vi "FRC Color Processing Example.vi"(0 "Image In":T1, 2 "LED Color":T5={"Hue"={110.52399131877658, 148.6727294921875}, "Sat"={34.78571428571429, 255.0}, "Val"={91.07142857142858, 255.0}} {"Hue" scale=0.0..255.0 scale format="%#_3g"}, 4 "Camera Type":T2=enum."MS HD3000 square") -> (7 "Original Image":T1(plugin-control), 9 "Detected Targets":T3(array[cluster]) {"Normalized Rect"."Numeric 5" format="%#_2g"; "Normalized Rect"."Numeric 3" format="%#_2g"; "Normalized Rect"."Numeric 2" format="%#_2g"; "Normalized Rect"."Numeric" format="%#_2g"})   [LabVIEW 2015]
uses:
  Users/allenpeters/git/Beachbot2016Dash/vision/Camera Types.ctl
  <vilib>/vision/Image Controls.llb/IMAQ Image.ctl
  <vilib>/vision/NI_Vision_Development_Module.lvlib
panel:
  in  "Std Devs for Calibration":cluster{"H":dbl, "S":dbl, "V":dbl}={"H"=4.0, "S"=6.0, "V"=6.0}
  out "Highest Avg Score":dbl format="%#_3g"
  in  "Min Score Threshold":i32=70
  in  "Emphasize Limit Tests":bool=TRUE
  in  "Aspect Ratio Fudge Factor":dbl=1.0
  in  "Annotation Limit":dbl=75.0
  in  "Annotate":bool=TRUE
  out "Sorted Particle Scores":T4(array[cluster]) {"Moment Factor" format="%#_3g"; "Aspect Ratio" format="%#_3g"; "Area to CH" format="%#_3g"; "X" format="%#_3g"; "Y" format="%#_3g"}
  out "Qualified Particles":i32
  out "Masked":T1(plugin-control)
  # "Instructions:\nUse Source to select image files from a directory, or use a USB or IP camera connected to your laptop.\nUse LED Color to threshold and build particles. Adjust HSV values to improve masking.\nClick and draw a line in Original Image to auto-calibrate to the LED color. You may need to widen Sat and Val.\nAnnotations draw a rectangle around \"good\" particles with scores from top to bottom."
  # "Density Profile"
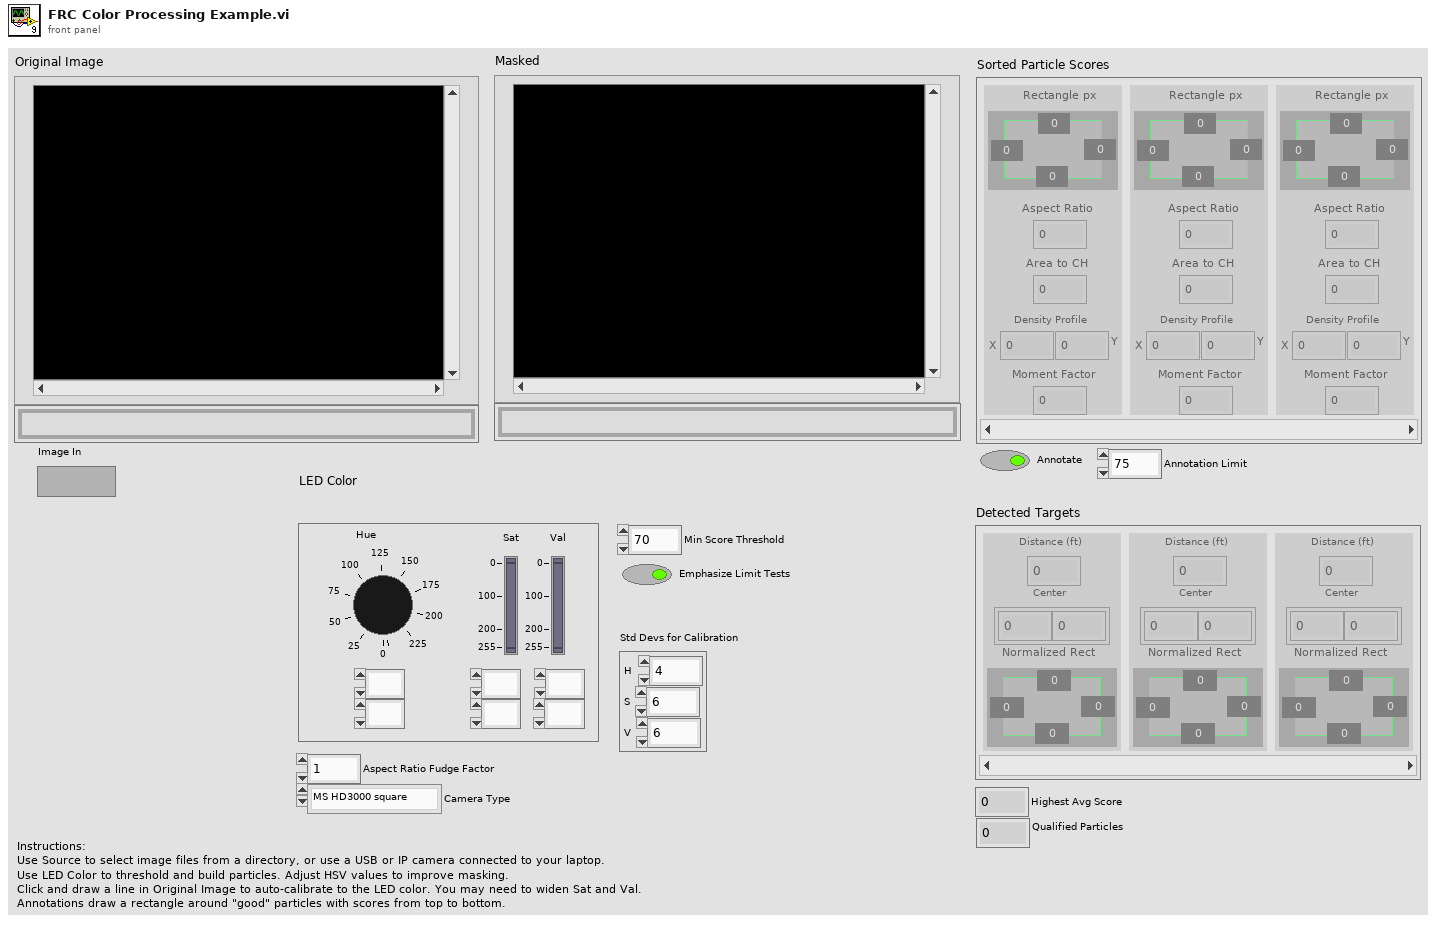
[diagram p1: front panel]
types:
  T1 = typedef "IMAQ Image.ctl" = refnum<image>
  T2 = typedef "Camera Types.ctl" = enum16{"206", "1011", "1013", "MS HD3000 square", "MS HD3000 640x480"}
  T3 = cluster{"Distance (ft)":dbl, "Center":cluster{dbl, dbl}, "Normalized Rect":cluster{"Numeric":dbl, "Numeric 2":dbl, "Numeric 3":dbl, "Numeric 5":dbl}}[]
  T4 = cluster{"Rectangle px":cluster{"Numeric":dbl, "Numeric 2":dbl, "Numeric 3":dbl, "Numeric 5":dbl}, "Aspect Ratio":dbl, "Area to CH":dbl, "X":dbl, "Y":dbl, "Moment Factor":dbl}[]
  T5 = cluster{"Hue":cluster{dbl, dbl}, "Sat":cluster{dbl, dbl}, "Val":cluster{dbl, dbl}}
  T6 = typedef "Particle Parameters" = i32
  T7 = typedef "Image Type" = u32
  T8 = cluster{cluster{dbl, dbl}, cluster{dbl, dbl}, cluster{dbl, dbl}}
  T9 = cluster{"Bounding box":cluster{"left":dbl, "top":dbl, "right":dbl, "bottom":dbl}, "Aspect Ratio":dbl, "Area to CH":dbl, "X Mask":dbl, "Y Mask":dbl, "Moment":dbl}[]
  T10 = cluster{"Rectangle":cluster{"Numeric":dbl, "Numeric 2":dbl, "Numeric 3":dbl, "Numeric 5":dbl}, "L":dbl, "Area to CH":dbl, "X":dbl, "Y":dbl, "Moment Factor":dbl}[]
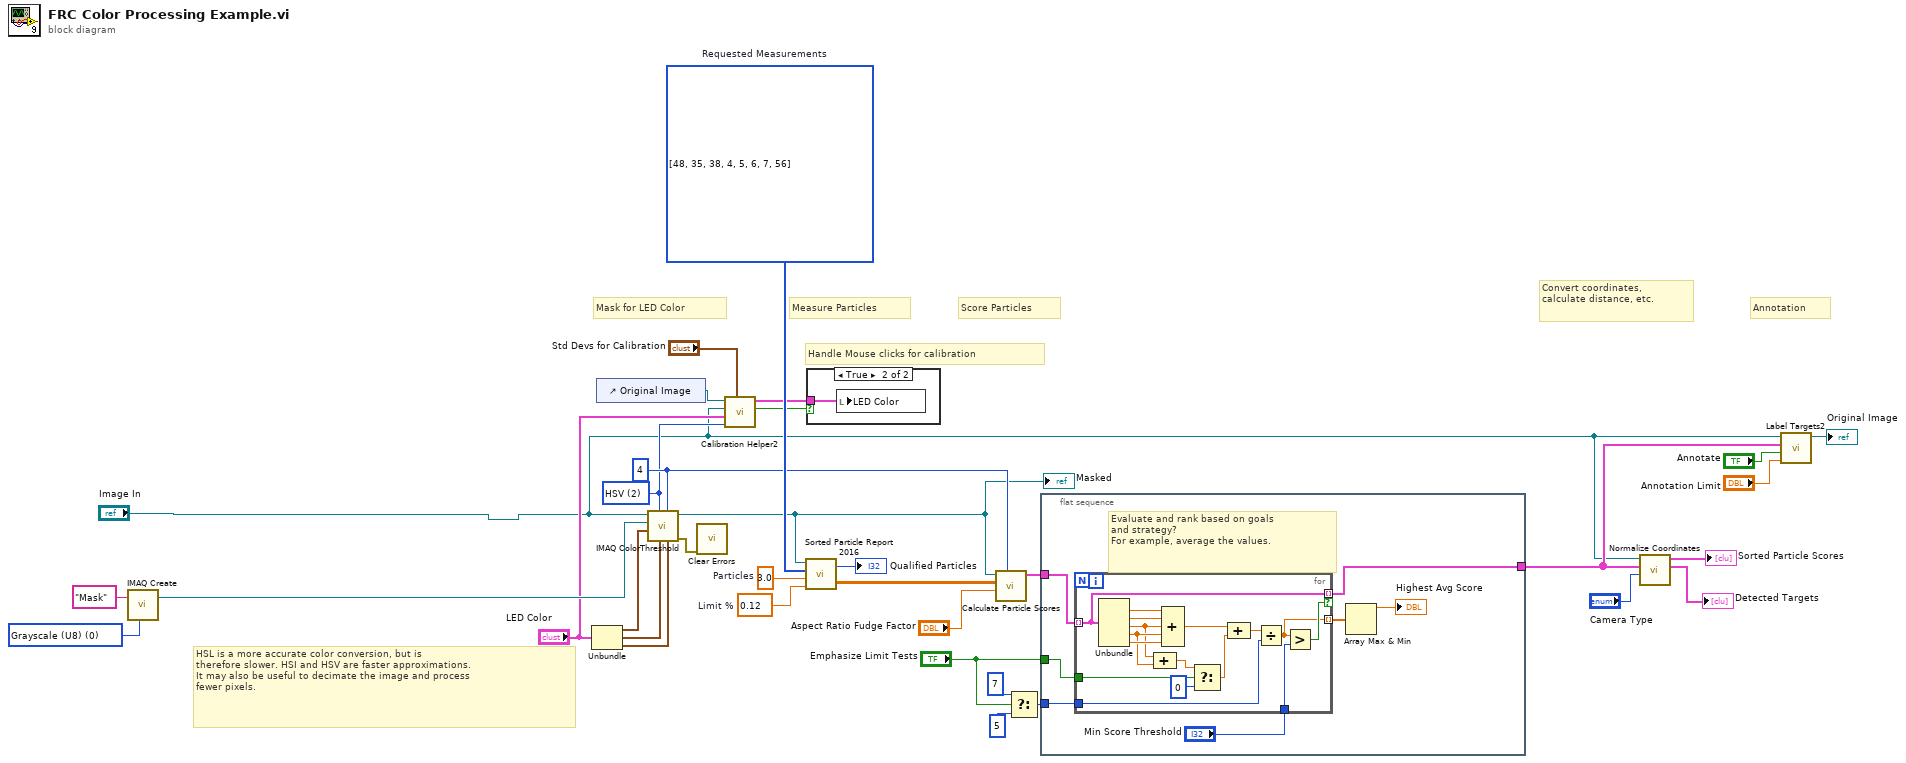
[diagram p0: block diagram]
diagram:
  w21 = 4 ("Replace Value")
  w24 = 0.12  # Limit %
  w27 = 3.0  # Particles
  w5 = u16 2 items=["RGB", "HSL", "HSV", "HSI"] ("Color Mode")
  w31 = T6[] [48, 35, 38, 4, 5, 6, 7, 56] items=["Center of Mass X", "Center of Mass Y", "First Pixel X", "First Pixel Y", "Bounding Rect Left", "Bounding Rect Top", "Bounding Rect Right", "Bounding Rect Bottom", "Max Feret Diameter Start X", "Max Feret Diameter Start Y", "Max Feret Diameter End X", "Max Feret Diameter End Y", "Max Horiz. Segment Length Left", "Max Horiz. Segment Length Right", "Max Horiz. Segment Length Row", "-", "Bounding Rect Width", "Bounding Rect Height", "Bounding Rect Diagonal", "Perimeter", "Convex Hull Perimeter", "Holes' Perimeter", "Max Feret Diameter", "Equivalent Ellipse Major Axis", "Equivalent Ellipse Minor Axis", "Equivalent Ellipse Minor Axis (Feret)", "Equivalent Rect Long Side", "Equivalent Rect Short Side", "Equivalent Rect Diagonal", "Equivalent Rect Short Side (Feret)", "Average Horiz. Segment Length", "Average Vert. Segment Length", "Hydraulic Radius", "Waddel Disk Diameter", "-", "Area", "Holes' Area", "Particle & Holes' Area", "Convex Hull Area", "Image Area", "-", "Number of Holes", "Number of Horiz. Segments", "Number of Vert. Segments", "-", "Orientation", "Max Feret Diameter Orientation", "-", "% Area/Image Area", "% Area/(Particle & Holes' Area)", "Ratio of Equivalent Ellipse Axes", "Ratio of Equivalent Rect Sides", "-", "Elongation Factor", "Compactness Factor", "Heywood Circularity Factor", "Type Factor", "-", "Sum X", "Sum Y", "Sum XX", "Sum XY", "Sum YY", "Sum XXX", "Sum XXY", "Sum XYY", "Sum YYY", "-", "Moment of Inertia XX", "Moment of Inertia XY", "Moment of Inertia YY", "Moment of Inertia XXX", "Moment of Inertia XXY", "Moment of Inertia XYY", "Moment of Inertia YYY", "Norm. Moment of Inertia XX", "Norm. Moment of Inertia XY", "Norm. Moment of Inertia YY", "Norm. Moment of Inertia XXX", "Norm. Moment of Inertia XXY", "Norm. Moment of Inertia XYY", "Norm. Moment of Inertia YYY", "Hu Moment 1", "Hu Moment 2", "Hu Moment 3", "Hu Moment 4", "Hu Moment 5", "Hu Moment 6", "Hu Moment 7"]  # Requested Measurements
  w34 = T7 0 items=["Grayscale (U8)", "Grayscale (I16)", "Grayscale (SGL)", "Complex (CSG)", "RGB (U32)", "HSL (U32)", "RGB (U64)", "Grayscale (U16)"] ("Image Type")
  # "Handle Mouse clicks for calibration"
  # "Measure Particles"
  # "Convert coordinates,\ncalculate distance, etc."
  # "Annotation"
  # "Score Particles"
  # "Mask for LED Color"
  # "HSL is a more accurate color conversion, but is\ntherefore slower. HSI and HSV are faster approximations.\nIt may also be useful to decimate the image and process\nfewer pixels."
  n1 = call "IMAQ Create"("Image Name"="Mask", "Image Type"=w34) -> ("New Image"=w32:T1)  [unwired: 2 in, 2 out]
  n2 = Unbundle("LED Color") -> ("Hue"=w30:cluster{dbl, dbl}, "Sat"=w29:cluster{dbl, dbl}, "Val"=w28:cluster{dbl, dbl})
  n3 = control-ref of="Original Image"() -> (w8:refnum<vi>)
  n4 = call "IMAQ ColorThreshold"("Blue or Luma or Val or Inten Range"=w28, "Replace Value"=w21, "Green or Sat Range"=w29, "Color Mode"=w5, "Red or Hue Range"=w30, "Image Dst"=w32, "Image Src"="Image In") -> ("error out"=w12:errorcluster, "Image Dst Out"=w13:T1)  [unwired: 3 in]
  "Masked" <- w13
  n5 = call <vilib>:"Clear Errors.vi"("error in (no error)"=w12) -> ()  [unwired: 5 in, 2 out]
  n6 = call "Calibration Helper2.vi"("Std Devs"="Std Devs for Calibration", "Color Mode"=w5, "Color Components"="LED Color", "Image"="Image In", "Image Ctl Refnum"=w8) -> ("Changed"=w7:bool, "output color"=w6:T8)  [unwired: 5 in]
  n7 = call "Sorted Particle Report 2016.vi"("Min Area Size %"=w24, "Particle Count Limit"=w27, "Pixel Measurements"=w31, "Image in"=w13) -> ("Sorted Data"=w25:dbl[][], "Particles"=→"Qualified Particles":i32)
  n8 = case shown="True" w7 {
    tunnel: w6 -> [_ w35]
    frame False {
    }
    frame True {
      n9 = local write "LED Color"(w35) -> ()
    }
  }
  n10 = call "Calculate Particle Scores.vi"("Pixel Value"=w21, "Aspect Fudge Factor"="Aspect Ratio Fudge Factor", "Sorted Data"=w25, "Image in"=w13) -> ("Scores"=w16:T9)  [unwired: 7 in]
  n11 = Select(t=7, s="Emphasize Limit Tests", f=5) -> (s? t:f=w9:i32)
  n12 = flat-sequence {
    tunnel: w16 -> [w41]
    tunnel: [w42] -> w14
    tunnel: w9 -> [w38]
    tunnel: "Emphasize Limit Tests" -> [w36]
    frame #0 {
      # "Evaluate and rank based on goals\nand strategy?\nFor example, average the values."
      n13 = for {
        tunnel: w41 -> [w56] mode=indexing
        tunnel: [w56] -> w42 mode=indexing if=w55
        tunnel: [w54] -> w40 mode=indexing
        tunnel: w38 -> [w53]
        tunnel: "Min Score Threshold" -> [w52]
        tunnel: w36 -> [w45]
        n14 = Unbundle(w56) -> ("Aspect Ratio"=w58:dbl, "Area to CH"=w57:dbl, "X Mask"=w47:dbl, "Y Mask"=w48:dbl, "Moment"=w49:dbl)  [unwired: 1 out]
        n15 = Compound Arithmetic op=ADD(w47, w48) -> (w46:dbl)
        n16 = Compound Arithmetic op=ADD(w58, w57, w47, w48, w49) -> (w51:dbl)
        n17 = Select(t=w46, s=w45, f=0) -> (s? t:f=w44:dbl)
        n18 = Compound Arithmetic op=ADD(w51, w44) -> (w50:dbl)
        n19 = Divide(x=w50, y=w53) -> (x/y=w54:dbl)
        n20 = Greater?(x=w54, y=w52) -> (0:w55:bool)
      }
      n21 = Array Max & Min(array=w40) -> (max value=→"Highest Avg Score":dbl)  [unwired: 3 out]
    }
  }
  n22 = call "Normalize Coordinates.vi"("Camera Type"="Camera Type", "Targets"=w14, "Image in"="Image In") -> ("Found Targets"=→"Detected Targets":T3, "Sorted Scores"=→"Sorted Particle Scores":T10)  [unwired: 7 in]
  n23 = call "Label Targets2.vi"("Score Threshold"="Annotation Limit", "Annotate"="Annotate", "Targets"=w14, "Image in"="Image In") -> ("Image out"=→"Original Image":T1)  [unwired: 7 in]
